vi "Holodrive.vi"(0 "Translation X":dbl, 5 "Translation Y":dbl, 7 "Angular":dbl, 9 "Robot Length":dbl=22.0, 11 "Robot Width":dbl=20.5) -> (2 "FL Rot":dbl, 3 "FR Rot":dbl, 4 "BL Rot":dbl, 6 "BR Rot":dbl, 10 "BR Drive":dbl, 13 "FL Drive":dbl, 14 "FR Drive":dbl, 15 "BL Drive":dbl)   [LabVIEW 2014]
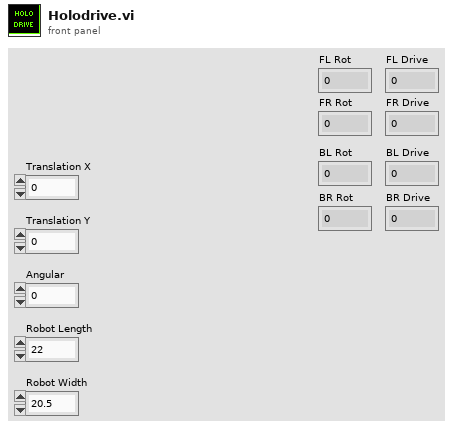
[diagram p1: front panel]
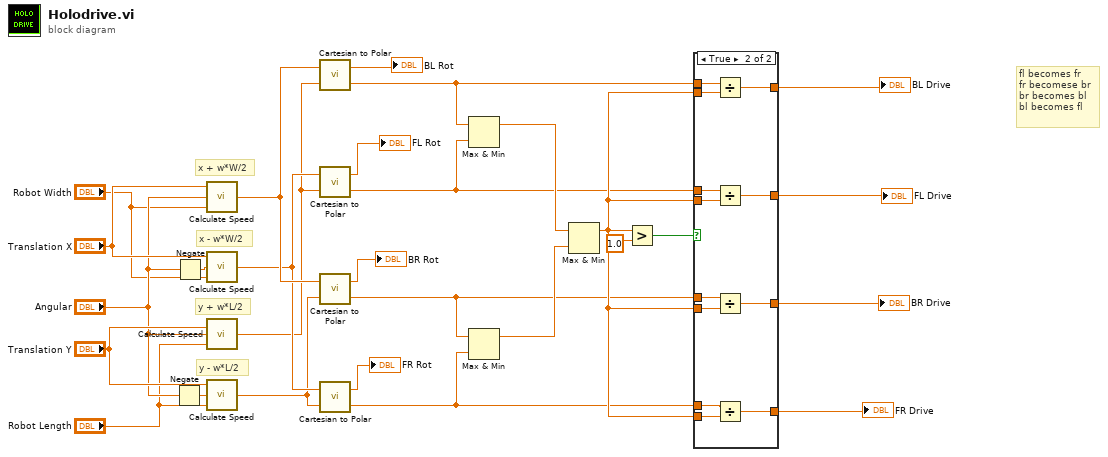
[diagram p0: block diagram]
diagram:
  # "fl becomes fr\nfr becomese br\nbr becomes bl\nbl becomes fl"
  # "y - w*L/2"
  # "y + w*L/2"
  # "x - w*W/2"
  # "x + w*W/2"
  n1 = Negate(x="Angular") -> (-x=w26:dbl)
  n2 = Negate(x="Angular") -> (-x=w25:dbl)
  n3 = call "Calculate Speed.vi"("dimension"="Robot Width", "rotational"="Angular", "translational"="Translation X") -> ("speed"=w16:dbl)
  n4 = call "Calculate Speed.vi"("dimension"="Robot Width", "rotational"=w25, "translational"="Translation X") -> ("speed"=w15:dbl)
  n5 = call "Calculate Speed.vi"("dimension"="Robot Length", "rotational"="Angular", "translational"="Translation Y") -> ("speed"=w14:dbl)
  n6 = call "Calculate Speed.vi"("dimension"="Robot Length", "rotational"=w26, "translational"="Translation Y") -> ("speed"=w13:dbl)
  n7 = call "Cartesian to Polar.vi"("y"=w14, "x"=w16) -> ("magnitude"=w12:dbl, "angle"=→"BL Rot":dbl)
  n8 = call "Cartesian to Polar.vi"("y"=w14, "x"=w15) -> ("magnitude"=w11:dbl, "angle"=→"FL Rot":dbl)
  n9 = call "Cartesian to Polar.vi"("y"=w13, "x"=w16) -> ("magnitude"=w10:dbl, "angle"=→"BR Rot":dbl)
  n10 = call "Cartesian to Polar.vi"("y"=w13, "x"=w15) -> ("magnitude"=w9:dbl, "angle"=→"FR Rot":dbl)
  n11 = Max & Min(x=w12, y=w11) -> (max(x,y)=w21:dbl)  [unwired: 1 out]
  n12 = Max & Min(x=w10, y=w9) -> (max(x,y)=w20:dbl)  [unwired: 1 out]
  n13 = Max & Min(x=w21, y=w20) -> (max(x,y)=w17:dbl)  [unwired: 1 out]
  n14 = Greater?(x=w17, y=1.0) -> (0:w18:bool)
  n15 = case shown="True" w18 {
    tunnel: w17 -> [_ w44]
    tunnel: w17 -> [_ w43]
    tunnel: w17 -> [_ w42]
    tunnel: w17 -> [_ w41]
    tunnel: [w32 w40] -> w4
    tunnel: [w31 w39] -> w3
    tunnel: [w30 w38] -> w2
    tunnel: [w29 w37] -> w1
    tunnel: w12 -> [w32 w36]
    tunnel: w11 -> [w31 w35]
    tunnel: w10 -> [w30 w34]
    tunnel: w9 -> [w29 w33]
    frame False {
    }
    frame True {
      n16 = Divide(x=w36, y=w41) -> (x/y=w40:dbl)
      n17 = Divide(x=w35, y=w42) -> (x/y=w39:dbl)
      n18 = Divide(x=w34, y=w43) -> (x/y=w38:dbl)
      n19 = Divide(x=w33, y=w44) -> (x/y=w37:dbl)
    }
  }
  "FL Drive" <- w3
  "FR Drive" <- w1
  "BL Drive" <- w4
  "BR Drive" <- w2
